vi "softwareXMLExpression.vi"(8 "postValue":string, 9 "preValue":string, 10 "xmlParser 0":string[](array[string]), 11 "String in":string) -> (1 "filter2":string, 2 "filter1":string, 3 "swXMLExpression":string)   [LabVIEW 2018]
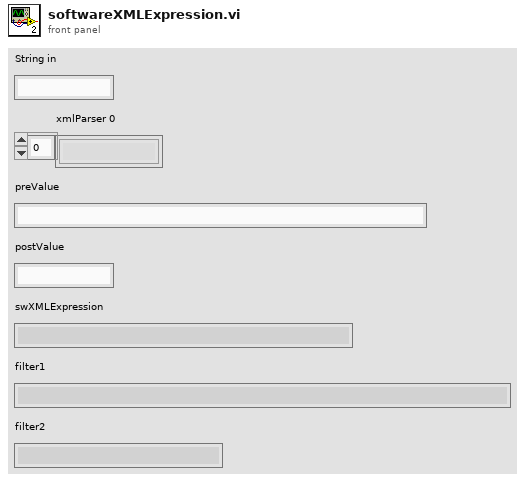
[diagram p1: front panel]
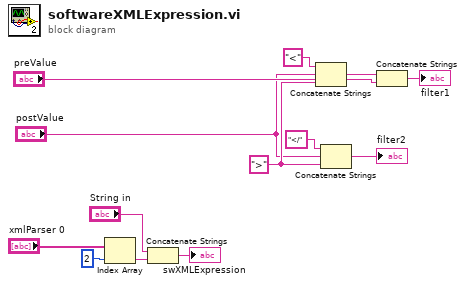
[diagram p0: block diagram]
diagram:
  w10 = ">" ("string")
  n1 = Index Array(array="xmlParser 0", index=2) -> (element=w3:string)
  n2 = Concatenate Strings("String in", w3) -> (→"swXMLExpression":string)
  n3 = Concatenate Strings("<" ("string"), "postValue", w10) -> (w12:string)
  n4 = Concatenate Strings("</" ("string"), "postValue", w10) -> (→"filter2":string)
  n5 = Concatenate Strings(w12, "preValue") -> (→"filter1":string)
